vi "Analog Write N Chans.vi"(7 "Analog Ref Override":dbl, 8 "Error In":errorcluster, 9 "AO Values":dbl[](array[numeric]), 10 "AO Channel(s)":u8[](array[numeric]), 11 "LINX Resource":T1) -> (0 "Error Out":errorcluster, 3 "LINX Resource":T1)   [LabVIEW 2013, in "LVH-LINX.lvlib"]
doc: "Write value(s) to the specified analog output channel(s)."
uses:
  <vilib>/LabVIEW Hacker/LINX/LVH-LINX.lvlib
  <vilib>/LabVIEW Hacker/LINX/Private/Type Defs/LINX Ref.ctl
  <vilib>/LabVIEW Hacker/LINX/Private/Type Defs/Platform.ctl
  <vilib>/LabVIEW Hacker/LINX/Private/Type Defs/Interface.ctl
  <vilib>/LabVIEW Hacker/LINX/Private/Device/Type Defs/LINX Device Config.ctl
  <vilib>/LabVIEW Hacker/LINX/Private/Device/Type Defs/TCP Config.ctl
  <vilib>/LabVIEW Hacker/LINX/Private/Type Defs/Device Family.ctl
  <vilib>/LabVIEW Hacker/LINX/Private/Type Defs/Peripheral.ctl
  <vilib>/LabVIEW Hacker/LINX/Private/myRIO/myRIO.lvlib
  <vilib>/LabVIEW Hacker/LINX/Private/Device/Device.lvlib
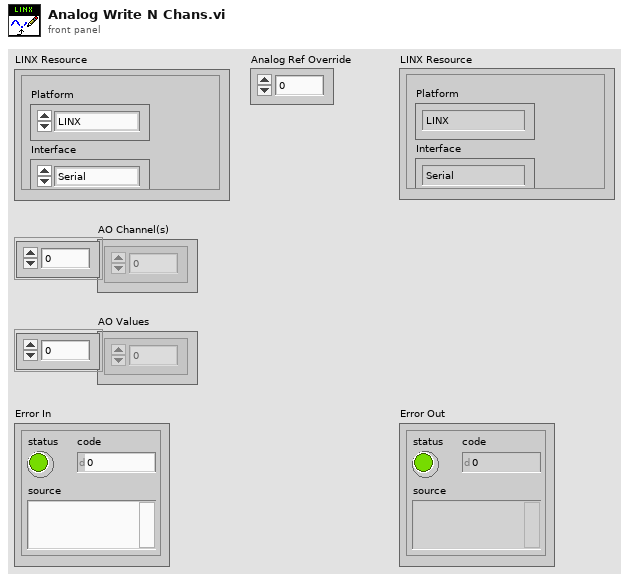
[diagram p1: front panel]
types:
  T1 = typedef "LVH-LINX.lvlib/LINX Ref.ctl" = cluster{"Platform":T2, "Interface":T3, "LINX Device Config":T4}
  T2 = typedef "LVH-LINX.lvlib/Platform.ctl" = enum16{"LINX", "myRIO"}
  T3 = typedef "LVH-LINX.lvlib/Interface.ctl" = enum16{"Serial", "TCP"}
  T4 = typedef "LVH-LINX.lvlib/Device.lvlib/LINX Device Config.ctl" = cluster{"Interface":T3, "COM Port":refnum<visa-resource-name>, "TCP Configuration":T5, "Device Family":T6, "Device ID":u8, "Device Name":string, "TCP Ref":refnum<k5>}
  T5 = typedef "LVH-LINX.lvlib/Device.lvlib/TCP Config.ctl" = cluster{"IP Address":string, "Port":u16}
  T6 = typedef "LVH-LINX.lvlib/Device Family.ctl" = enum8{"National Instruments", "Digilent", "Arduino"}
  T7 = typedef "LVH-LINX.lvlib/Peripheral.ctl" = enum8{"DI", "DO", "AI", "AO", "PWM", "QE", "UART", "I2C", "SPI", "CAN"}
  T8 = typedef "AO.lvlib/AO Reference.ctl" = cluster{"myRIO Reference":T9, "AO Channel List":T13, "AO Scaling Constant List":T15}
  T9 = typedef "myRIO Generic Hardware Reference.ctl" = cluster{"myRIO Model":T10, "myRIO Hardware Reference":T11}
  T10 = typedef "Hardware Version Enum.ctl" = enum16{"Unknown", "myRIO-1900", "myRIO-1950"}
  T11 = typedef "myRIO v1.0 Reference.ctl" = cluster{"Generic FPGA Reference":T12, "Allow multiple opens":bool}
  T12 = typedef "Generic FPGA Reference.ctl" = refnum<k20>
  T13 = typedef "AO Channels List.ctl" = T14[]
  T14 = typedef "AO Channels Enum.ctl" = enum16{"Not Connected", "AudioOut/Left", "AudioOut/Right", "C/AO0", "C/AO1", "A/AO0", "A/AO1", "B/AO0", "B/AO1"}
  T15 = typedef "Analog Scaling Constants List.ctl" = T16[]
  T16 = typedef "Analog Scaling Constants.ctl" = cluster{"LSB Weight (Volts)":dbl, "Offset (Volts)":dbl, "Signed?":bool}
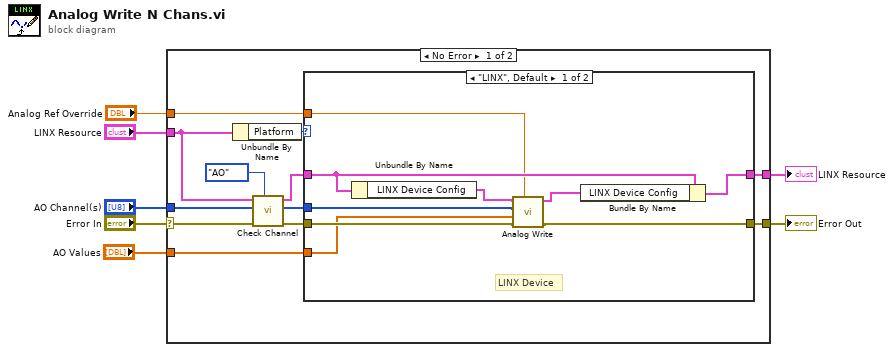
[diagram p0: block diagram]
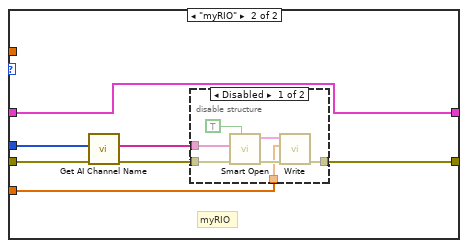
[diagram p2: hidden frame]
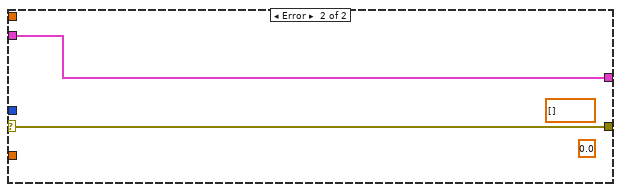
[diagram p4: hidden frame]
diagram:
  n1 = case shown="No Error" "Error In" {
    selector: "Error In" -> [w9 w45]
    tunnel: [w18 w45] -> w7
    tunnel: [w17 w44] -> w6
    tunnel: "LINX Resource" -> [w12 w44]
    tunnel: "AO Channel(s)" -> [w11 _]
    tunnel: "Analog Ref Override" -> [w10 _]
    tunnel: "AO Values" -> [w8 _]
    frame No Error {
      n2 = Unbundle By Name(w12) -> ("Platform"=w19:T2)
      n3 = call <vilib>:"Check Channel.vi"("Peripheral"=Peripheral."AO", "Error In"=w9, "Channels"=w11, "LINX Resource"=w12) -> ("Error Out"=w16:errorcluster, "Channels"=w15:u8[], "LINX Resource"=w13:T1)  [unwired: 5 in]
      n4 = case shown="\"LINX\", Default" w19 {
        tunnel: w16 -> [w23 w31]
        tunnel: w13 -> [w28 w35]
        tunnel: [w24 w33] -> w18
        tunnel: [w27 w35] -> w17
        tunnel: w15 -> [w22 w34]
        tunnel: w10 -> [w20 _]
        tunnel: w8 -> [w21 w29]
        frame "LINX", Default {
          # "LINX Device"
          n5 = Unbundle By Name(w28) -> ("LINX Device Config"=w26:T4)
          n6 = call <vilib>:"Analog Write.vi"("Analog Ref Override"=w20, "Error In"=w23, "AO Values"=w21, "AO Channels"=w22, "LINX Device Config"=w26) -> ("Error Out"=w24:errorcluster, "LINX Device Config"=w25:T4)  [unwired: 5 in]
          n7 = Bundle By Name(cluster=w28, "LINX Device Config"=w25) -> (w27:T1)
        }
        frame "myRIO" {
          # "myRIO"
          n8 = call <vilib>:"Get AI Channel Name.vi"("Error In"=w31, "AI Channel Nums"=w34) -> ("Error Out"=w30:errorcluster, "AI Channels"=w32:string[])  [unwired: 7 in]
          n9 = disable-structure shown="Disabled" {
            disable-tunnel: w30 -> [w39 w43]
            disable-tunnel: [w37 w43] -> w33
            disable-tunnel: w32 -> [w38 _]
            disable-tunnel: w29 -> [w36 _]
            frame Disabled {
              n10 = call <vilib>:"Smart Open.vi"("Allow multiple opens?"=TRUE, "error in (no error)"=w39, "Channel Names"=w38) -> ("error out"=w41:errorcluster, "AO Ref Out"=w42:T8)  [unwired: 7 in]
              n11 = call <vilib>:"Write.vi"("error in (no error)"=w41, "Values"=w36, "AO Ref In"=w42) -> ("error out"=w37:errorcluster)  [unwired: 6 in, 1 out]
            }
            frame Enabled {
            }
          }
        }
      }
    }
    frame Error {
      (unwired) 0.0 ("AI Ref")
      (unwired) dbl[] [] ("Values")
    }
  }
  "Error Out" <- w7
  "LINX Resource" <- w6
